vi "Process.vi"(8 "error in (no error)":errorcluster, 11 "Execution API In":refnum<class "Execution API.lvclass">) -> (0 "error out":errorcluster, 3 "Execution API Out":refnum<class "Execution API.lvclass">)   [LabVIEW 2020, in "Execution API.lvclass"]
uses:
  Execution API.lvclass
  Execution API.lvclass/Execution API.ctl
  Application Framework/Process Classes/Process/Process.lvclass
  <vilib>/ErrorRing/Error Ring.xnode
  Helper Classes/Test Finder/Test Finder.lvclass
  Test Runner/Test Runner.lvclass
  Report Generator/Report Generator.lvclass
  Helper Classes/Project Loader/Project Loader.lvclass
  Test Suite/LUnit Test Suite.lvclass
  C:/Git/astemes-lunit/source/Application Framework/Process Classes/Process/Process.lvclass
  C:/Git/astemes-lunit/source/Framework/Execution API/Execution API.lvclass
  C:/Git/astemes-lunit/source/Framework/Test Runner/Test Runner.lvclass
  C:/Git/astemes-lunit/source/Framework/Report Generator/Report Generator.lvclass
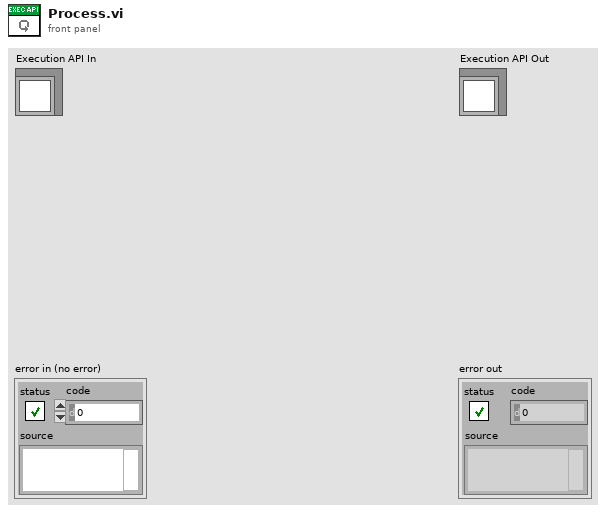
[diagram p1: front panel]
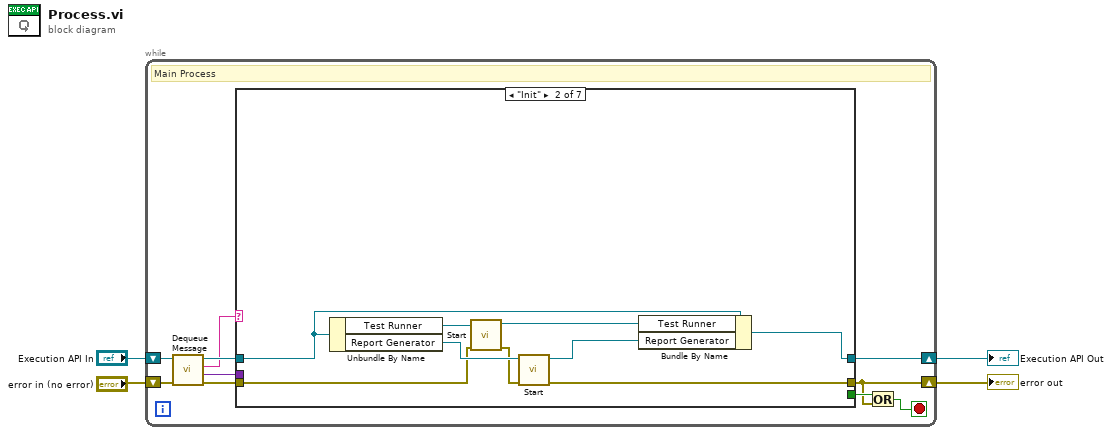
[diagram p0: block diagram]
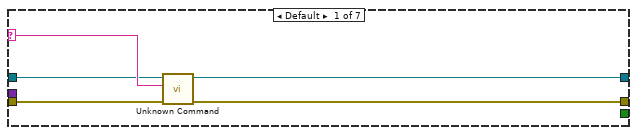
[diagram p2: hidden frame]
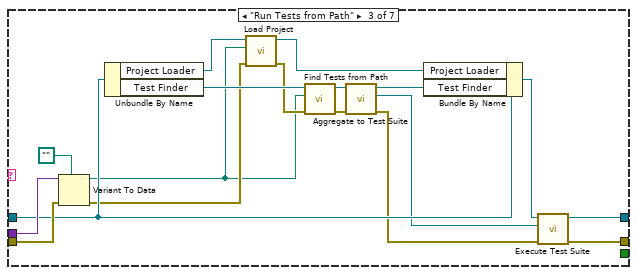
[diagram p3: hidden frame]
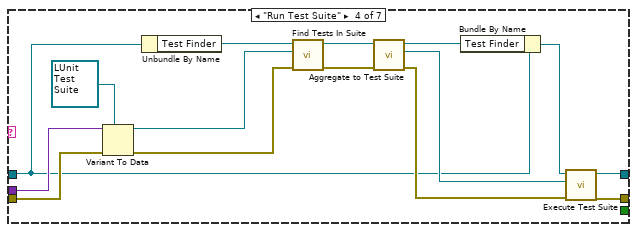
[diagram p4: hidden frame]
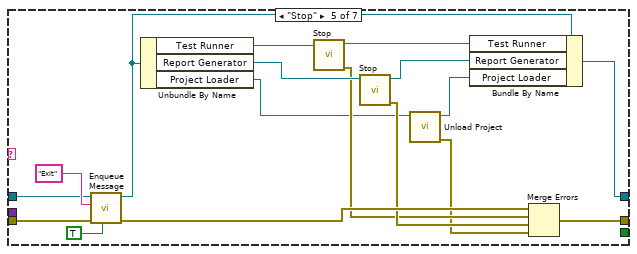
[diagram p5: hidden frame]
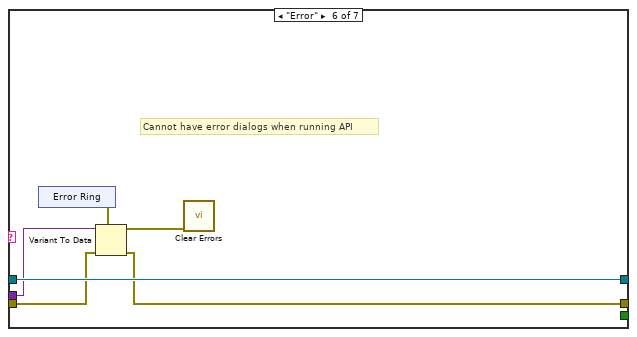
[diagram p6: hidden frame]
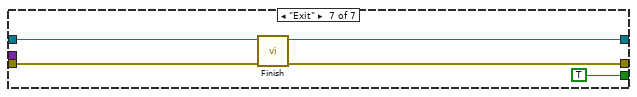
[diagram p7: hidden frame]
diagram:
  n1 = while {
    shift-right: [w6] -> w4
    shift-left: "error in (no error)" -> [w13]
    shift-right: [w5] -> w3
    shift-left: "Execution API In" -> [w14]
    stop <- w7 stop-if-true
    # "Main Process"
    n2 = call "Dequeue Message.vi"("error in (no error)"=w13, "Process In"=w14) -> ("error out"=w12:errorcluster, "Message Data"=w9:variant, "Message"=w10:string, "Process Out"=w11:refnum<class "Execution API.lvclass">)  [unwired: 6 in]
    n3 = case shown="\"Init\"" w10 {
      selector: w10 -> [w19 _ _ _ _ _ _]
      tunnel: [w16 w20 w32 w50 w69 w80 w87] -> w6
      tunnel: w12 -> [w15 w26 w46 w60 w70 w83 w86]
      tunnel: [w18 w21 w31 w51 w73 w84 w88] -> w5
      tunnel: w11 -> [w17 w22 w43 w49 w71 w84 w89]
      tunnel: w9 -> [_ _ w45 w61 _ w82 _]
      tunnel: [_ _ _ _ _ _ TRUE] -> w8
      frame Default {
        n4 = call "Unknown Command.vi"("error in (no error)"=w15, "String"=w19, "Process In"=w17) -> ("error out"=w16:errorcluster, "Process Out"=w18:refnum<class "Execution API.lvclass">)  [unwired: 7 in]
      }
      frame "Init" {
        n5 = Unbundle By Name(w22) -> ("Test Runner"=w28:refnum<class "Test Runner.lvclass">, "Report Generator"=w27:refnum<class "Report Generator.lvclass">)
        n6 = call "Start.vi"("error in (no error)"=w26, "Process In"=w28) -> ("error out"=w25:errorcluster, "Process Out"=w24:refnum<class "Test Runner.lvclass">)  [unwired: 8 in]
        n7 = call "Start.vi"("error in (no error)"=w25, "Process In"=w27) -> ("error out"=w20:errorcluster, "Process Out"=w23:refnum<class "Report Generator.lvclass">)  [unwired: 8 in]
        n8 = Bundle By Name(cluster=w22, "Test Runner"=w24, "Report Generator"=w23) -> (w21:refnum<class "Execution API.lvclass">)
      }
      frame "Run Tests from Path" {
        n9 = Variant To Data(error in=w46, type=path "", Variant=w45) -> (data=w38:path, error out=w39:errorcluster)
        n10 = Unbundle By Name(w43) -> ("Project Loader"=w41:refnum<class "Project Loader.lvclass">, "Test Finder"=w42:refnum<class "Test Finder.lvclass">)
        n11 = call "Load Project.vi"("error in (no error)"=w39, "Project or Class Path"=w38, "Project Loader In"=w41) -> ("error out"=w40:errorcluster, "Project Loader Out"=w37:refnum<class "Project Loader.lvclass">)  [unwired: 7 in]
        n12 = call-dynamic "Find Tests from Path.vi"("error in (no error)"=w40, "Project or Class Path"=w38, "Test Case Finder In"=w42) -> ("error out"=w34:errorcluster, "Test Case Finder Out"=w36:refnum<class "Test Finder.lvclass">)  [unwired: 7 in]
        n13 = call "Aggregate to Test Suite.vi"("error in (no error)"=w34, "Test Finder In"=w36) -> ("error out"=w33:errorcluster, "Test Suite"=w30:refnum<class "LUnit Test Suite.lvclass">, "Test Finder Out"=w35:refnum<class "Test Finder.lvclass">)  [unwired: 7 in]
        n14 = Bundle By Name(cluster=w43, "Project Loader"=w37, "Test Finder"=w35) -> (w29:refnum<class "Execution API.lvclass">)
        n15 = call "Execute Test Suite.vi"("error in (no error)"=w33, "Test Suite"=w30, "Execution API in"=w29) -> ("error out"=w32:errorcluster, "Execution API out"=w31:refnum<class "Execution API.lvclass">)  [unwired: 7 in]
      }
      frame "Run Test Suite" {
        n16 = Variant To Data(error in=w60, type=refnum<class "LUnit Test Suite.lvclass"> refnum ("Test Case"), Variant=w61) -> (data=w47:refnum<class "LUnit Test Suite.lvclass">, error out=w48:errorcluster)
        n17 = Unbundle By Name(w49) -> ("Test Finder"=w58:refnum<class "Test Finder.lvclass">)
        n18 = call "Find Tests In Suite.vi"("error in (no error)"=w48, "Test Suite"=w47, "Test Finder In"=w58) -> ("error out"=w55:errorcluster, "Test Finder Out"=w57:refnum<class "Test Finder.lvclass">)  [unwired: 7 in]
        n19 = call "Aggregate to Test Suite.vi"("error in (no error)"=w55, "Test Finder In"=w57) -> ("error out"=w54:errorcluster, "Test Suite"=w53:refnum<class "LUnit Test Suite.lvclass">, "Test Finder Out"=w56:refnum<class "Test Finder.lvclass">)  [unwired: 7 in]
        n20 = Bundle By Name(cluster=w49, "Test Finder"=w56) -> (w52:refnum<class "Execution API.lvclass">)
        n21 = call "Execute Test Suite.vi"("error in (no error)"=w54, "Test Suite"=w53, "Execution API in"=w52) -> ("error out"=w50:errorcluster, "Execution API out"=w51:refnum<class "Execution API.lvclass">)  [unwired: 7 in]
      }
      frame "Stop" {
        n22 = call "Enqueue Message.vi"("Priority Message? (F)"=TRUE, "error in (no error)"=w70, "Message"="Exit", "Process In"=w71) -> ("error out"=w68:errorcluster, "Process Out"=w72:refnum<class "Execution API.lvclass">)  [unwired: 6 in]
        n23 = Unbundle By Name(w72) -> ("Test Runner"=w78:refnum<class "Test Runner.lvclass">, "Report Generator"=w77:refnum<class "Report Generator.lvclass">, "Project Loader"=w64:refnum<class "Project Loader.lvclass">)
        n24 = call-dynamic "Stop.vi"("Test Runner In"=w78) -> ("error out"=w66:errorcluster, "Test Runner Out"=w76:refnum<class "Test Runner.lvclass">)  [unwired: 8 in, 1 out]
        n25 = call-dynamic "Stop.vi"("Process In"=w77) -> ("error out"=w67:errorcluster, "Process Out"=w75:refnum<class "Report Generator.lvclass">)  [unwired: 8 in, 1 out]
        n26 = call "Unload Project.vi"("Project Loader In"=w64) -> ("error out"=w62:errorcluster, "Project Loader Out"=w63:refnum<class "Project Loader.lvclass">)  [unwired: 9 in]
        n27 = Bundle By Name(cluster=w72, "Test Runner"=w76, "Report Generator"=w75, "Project Loader"=w63) -> (w73:refnum<class "Execution API.lvclass">)
        n28 = Merge Errors(w68, w66, w67, w62) -> (w69:errorcluster)
      }
      frame "Error" {
        # "Cannot have error dialogs when running API"
        n29 = xnode "Error Ring"() -> ("error out"=w81:errorcluster)
        n30 = Variant To Data(error in=w83, type=w81, Variant=w82) -> (data=w79:errorcluster, error out=w80:errorcluster)
        n31 = call <vilib>:"Clear Errors.vi"("error in (no error)"=w79) -> ()  [unwired: 5 in, 2 out]
      }
      frame "Exit" {
        n32 = call "Finish.vi"("error in (no error)"=w86, "Process In"=w89) -> ("error out"=w87:errorcluster, "Process Out"=w88:refnum<class "Execution API.lvclass">)  [unwired: 8 in]
      }
    }
    n33 = Or(x=w8, y=w6) -> (x .or. y?=w7:bool)
  }
  "error out" <- w4
  "Execution API Out" <- w3
